vi "Test Dequeue Element.vi"() -> ()   [LabVIEW 2013]
uses:
  <vilib>/addons/_JKI Toolkits/Caraya/classes/Assert/Assert True.vi
  Circular Buffers/ByteFIFO/ByteFIFO.lvclass
  Circular Buffers/VariantBuffer/VariantBuffer.lvclass
  <vilib>/addons/_JKI Toolkits/Caraya/classes/Assert/Assert.lvclass
  <vilib>/addons/_JKI Toolkits/Caraya/classes/Test/Test.lvclass
panel:
  out "overflow 2":u8[](array[numeric]) format="%02x"
  out "dequeued 2":u8[](array[numeric]) format="%02x"
  out "index2 byte 2":u8 format="%02x"
  out "index2 byte":u8 format="%02x"
  out "dequeued":u8[](array[numeric]) format="%02x"
  out "overflow":u8[](array[numeric]) format="%02x"
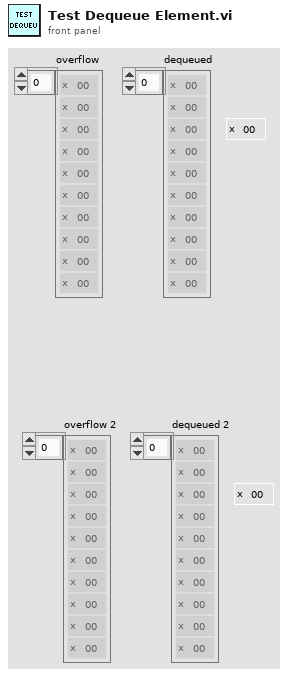
[diagram p1: front panel]
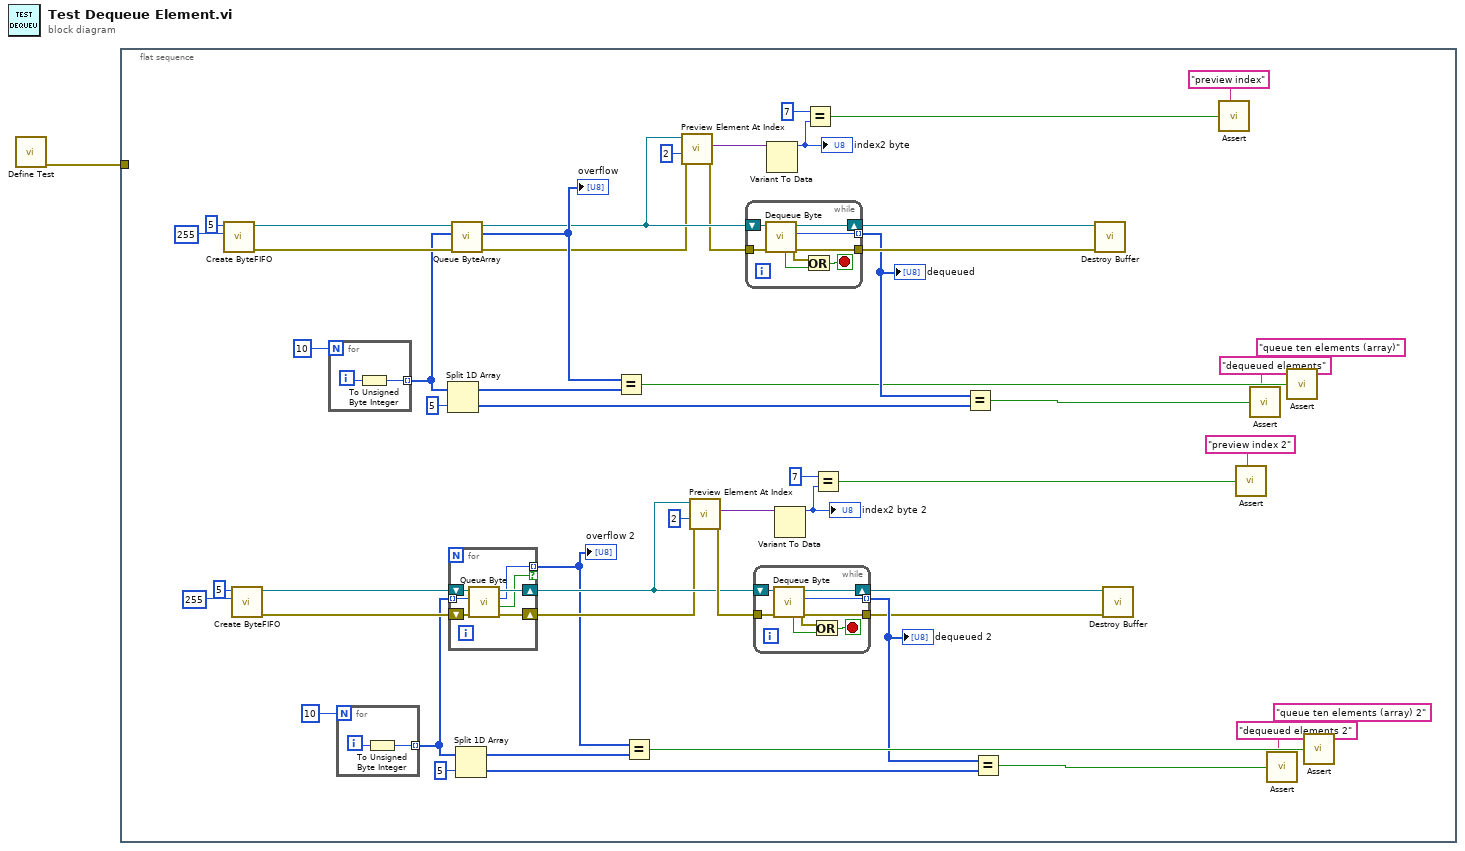
[diagram p0: block diagram]
diagram:
  n1 = call <vilib>:"Define Test.vi"() -> ("error out"=w1:errorcluster)  [unwired: 10 in, 1 out]
  n2 = flat-sequence {
    tunnel: w1 -> [_]
    frame #0 {
      n3 = call "Create ByteFIFO.vi"("default value"=u8 255, "bufSize"=5) -> ("error out"=w50:errorcluster, "Buffer"=w51:refnum<data-value>)  [unwired: 8 in]
      n4 = call "Create ByteFIFO.vi"("default value"=u8 255, "bufSize"=5) -> ("error out"=w11:errorcluster, "Buffer"=w13:refnum<data-value>)  [unwired: 8 in]
      n5 = for {
        N: 10 -> [_]
        tunnel: [w70] -> w45 mode=indexing
        i -> [w71]
        n6 = To Unsigned Byte Integer(number=w71) -> (unsigned 8bit integer=w70:u8)
      }
      n7 = for {
        N: 10 -> [_]
        tunnel: [w61] -> w9 mode=indexing
        i -> [w62]
        n8 = To Unsigned Byte Integer(number=w62) -> (unsigned 8bit integer=w61:u8)
      }
      n9 = Split 1D Array(array=w45, index=5) -> (first subarray=w43:u8[], second subarray=w42:u8[])
      n10 = for {
        tunnel: w9 -> [w56] mode=indexing
        tunnel: [w55] -> w8 mode=indexing if=w54
        shift-right: [w59] -> w12
        shift-left: w13 -> [w60]
        shift-right: [w57] -> w10
        shift-left: w11 -> [w58]
        n11 = call "Queue Byte.vi"("error in"=w58, "byte"=w56, "Buffer"=w60) -> ("error out"=w57:errorcluster, "overflowed?"=w54:bool, "overflow"=w55:u8, "Buffer"=w59:refnum<data-value>)  [unwired: 5 in]
      }
      "overflow 2" <- w8
      n12 = call "Queue ByteArray.vi"("error in"=w50, "bytes"=w45, "Buffer"=w51) -> ("error out"=w40:errorcluster, "overflow"=w46:u8[], "Buffer"=w41:refnum<data-value>)  [unwired: 6 in]
      "overflow" <- w46
      n13 = Split 1D Array(array=w9, index=5) -> (first subarray=w20:u8[], second subarray=w21:u8[])
      n14 = Equal?(x=w46, y=w43) -> (x = y?=w33:bool)
      n15 = Equal?(x=w8, y=w20) -> (x = y?=w28:bool)
      n16 = call "Preview Element At Index.vi"("error in"=w40, "index"=2 ("index (-1: last)"), "Buffer in"=w41) -> ("error out"=w39:errorcluster, "element"=w37:variant)  [unwired: 5 in, 2 out]
      n17 = call "Preview Element At Index.vi"("error in"=w10, "index"=2 ("index (-1: last)"), "Buffer in"=w12) -> ("error out"=w22:errorcluster, "element"=w24:variant)  [unwired: 5 in, 2 out]
      n18 = while {
        tunnel: w39 -> [w76]
        tunnel: [w74] -> w47
        tunnel: [w75] -> w34 mode=indexing
        shift-right: [w77] -> w48
        shift-left: w41 -> [w78]
        stop <- w73 stop-if-true
        n19 = call "Dequeue Byte.vi"("error in"=w76, "Buffer"=w78) -> ("error out"=w74:errorcluster, "byte"=w75:u8, "Buffer"=w77:refnum<data-value>, "buffer empty?"=w72:bool)  [unwired: 5 in, 1 out]
        n20 = Or(x=w74, y=w72) -> (x .or. y?=w73:bool)
      }
      "dequeued" <- w34
      n21 = while {
        tunnel: w22 -> [w67]
        tunnel: [w65] -> w18
        tunnel: [w66] -> w27 mode=indexing
        shift-right: [w68] -> w17
        shift-left: w12 -> [w69]
        stop <- w64 stop-if-true
        n22 = call "Dequeue Byte.vi"("error in"=w67, "Buffer"=w69) -> ("error out"=w65:errorcluster, "byte"=w66:u8, "Buffer"=w68:refnum<data-value>, "buffer empty?"=w63:bool)  [unwired: 5 in, 1 out]
        n23 = Or(x=w65, y=w63) -> (x .or. y?=w64:bool)
      }
      "dequeued 2" <- w27
      n24 = Variant To Data(Variant=w37) -> (data=w36:u8)  [unwired: 2 in, 1 out]
      "index2 byte" <- w36
      n25 = Variant To Data(Variant=w24) -> (data=w25:u8)  [unwired: 2 in, 1 out]
      "index2 byte 2" <- w25
      n26 = Equal?(x=u8 7, y=w36) -> (x = y?=w31:bool)
      n27 = Equal?(x=u8 7, y=w25) -> (x = y?=w30:bool)
      n28 = Equal?(x=w34, y=w42) -> (x = y?=w32:bool)
      n29 = Equal?(x=w27, y=w21) -> (x = y?=w29:bool)
      n30 = call "Destroy Buffer.vi"("error in"=w47, "Buffer"=w48) -> ()  [unwired: 8 in, 2 out]
      n31 = call "Destroy Buffer.vi"("error in"=w18, "Buffer"=w17) -> ()  [unwired: 8 in, 2 out]
      n32 = call-poly <vilib>:"Assert.vi"("Label"="preview index", "True?"=w31) -> ()  [unwired: 8 in, 2 out]
      n33 = call-poly <vilib>:"Assert.vi"("Label"="preview index 2", "True?"=w30) -> ()  [unwired: 8 in, 2 out]
      n34 = call-poly <vilib>:"Assert.vi"("Label"="dequeued elements", "True?"=w32) -> ()  [unwired: 8 in, 2 out]
      n35 = call-poly <vilib>:"Assert.vi"("Label"="dequeued elements 2", "True?"=w29) -> ()  [unwired: 8 in, 2 out]
      n36 = call-poly <vilib>:"Assert.vi"("Label"="queue ten elements (array)", "True?"=w33) -> ()  [unwired: 8 in, 2 out]
      n37 = call-poly <vilib>:"Assert.vi"("Label"="queue ten elements (array) 2", "True?"=w28) -> ()  [unwired: 8 in, 2 out]
    }
  }
